vi "init-vr-scene-window.vi"(8 "错误输入（无错误）":errorcluster, 11 "SceneWindow输入":refnum<vi>) -> (0 "错误输出":errorcluster, 3 "SceneWindow输出":refnum<vi>)   [LabVIEW 2013]
uses:
  <vilib>/Utility/miscctls.llb/LVRectTypeDef.ctl
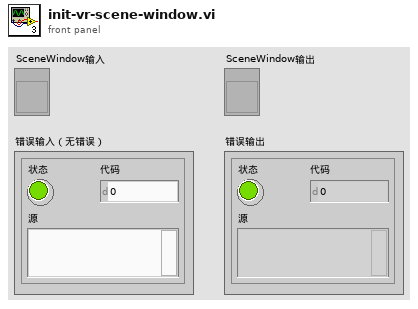
[diagram p1: front panel]
types:
  T1 = enum16{"Open", "Minimized", "Maximized", "Hidden"}
  T2 = typedef "LVRectTypeDef.ctl" = cluster{"Left":i16, "Top":i16, "Right":i16, "Bottom":i16}
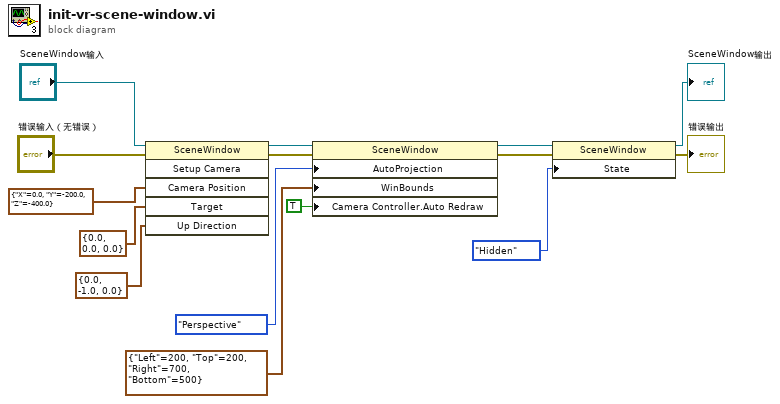
[diagram p0: block diagram]
diagram:
  n1 = invoke class="SceneWindow" method="Setup Camera"(reference="SceneWindow输入", error in="错误输入（无错误）", "Camera Position"=cluster{"X":sgl, "Y":sgl, "Z":sgl} {"X"=0.0, "Y"=-200.0, "Z"=-400.0}, "Target"=cluster{"X":sgl, "Y":sgl, "Z":sgl} {"X"=0.0, "Y"=0.0, "Z"=0.0}, "Up Direction"=cluster{"X":sgl, "Y":sgl, "Z":sgl} {"X"=0.0, "Y"=-1.0, "Z"=0.0}) -> (reference out=w11:refnum<vi>, error out=w7:errorcluster)  [unwired: 1 in, 4 out]
  n2 = property class="SceneWindow"(reference=w11, error in=w7, "AutoProjection"=enum16{"None", "Perspective", "Orthographic"}."Perspective" ("Automatic Projection Mode"), "WinBounds"=T2 {"Left"=200, "Top"=200, "Right"=700, "Bottom"=500} ("Window Bounds"), "Camera Controller.Auto Redraw"=TRUE ("Camera Controller:Auto Redraw")) -> (reference out=w8:refnum<vi>, error out=w6:errorcluster)
  n3 = property class="SceneWindow"(reference=w8, error in=w6, "State"=T1."Hidden" ("Window State")) -> (reference out=→"SceneWindow输出":refnum<vi>, error out=→"错误输出":errorcluster)
